vi "MakeFolderInSystemDirectry.vi"(8 "エラー入力（エラーなし）":errorcluster, 10 "名前または相対パス":string, 11 "system directory type":T1 items=["User Home"=0, "User Desktop"=1, "User Documents"=2, "User Application Data"=3, "User Preferences"=4, "User Temporary"=5, "Public Documents"=6, "Public Application Data"=7, "Public Preferences"=8, "Public Cache"=13, "System Core Libraries"=9, "System Installed Libraries"=10, "Application Files"=11, "Boot Volume Root"=12]) -> (0 "エラー出力":errorcluster, 3 "dup path":path)   [LabVIEW 2021]
uses:
  <vilib>/Utility/sysdir.llb/System Directory Type.ctl
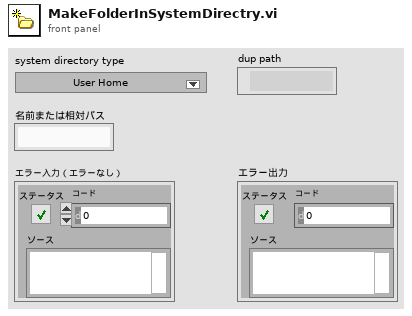
[diagram p1: front panel]
types:
  T1 = typedef "System Directory Type.ctl" = i32
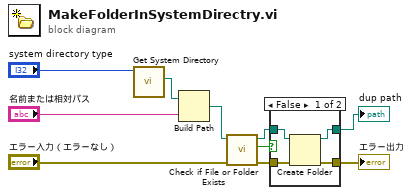
[diagram p0: block diagram]
diagram:
  n1 = call <vilib>:"Get System Directory.vi"("system directory type"="system directory type") -> ("system directory"=w2:path)  [unwired: 10 in]
  n2 = Build Path(base path=w2, name or relative path="名前または相対パス") -> (appended path=w4:path)
  n3 = call <vilib>:"Check if File or Folder Exists.vi"("error in (no error)"="エラー入力（エラーなし）", "path"=w4) -> ("error out"=w7:errorcluster, "file or folder exists?"=w5:bool, "dup path"=w6:path)  [unwired: 7 in]
  n4 = case shown="False" w5 {
    tunnel: w6 -> [w14 w15]
    tunnel: [w13 w15] -> w9
    tunnel: w7 -> [w12 w16]
    tunnel: [w11 w16] -> w10
    frame False {
      n5 = Create Folder(path (use dialog)=w14, error in=w12) -> (created path=w13:path, error out=w11:errorcluster)  [unwired: 1 in, 1 out]
    }
    frame True {
    }
  }
  "エラー出力" <- w10
  "dup path" <- w9
